vi "ChooseCowlState.vi"(0 "Distance":dbl) -> (1 "A,B,C":string)   [LabVIEW 2019]
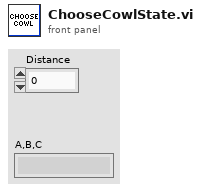
[diagram p1: front panel]
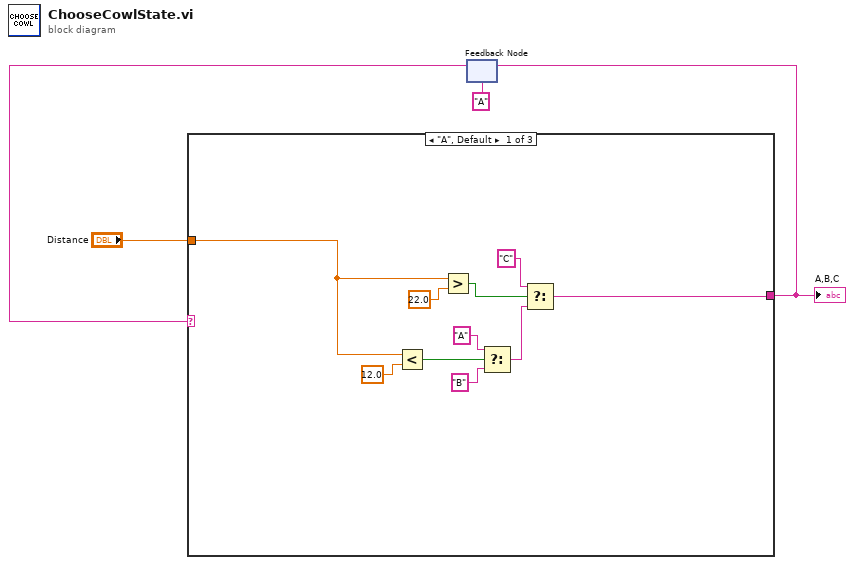
[diagram p0: block diagram]
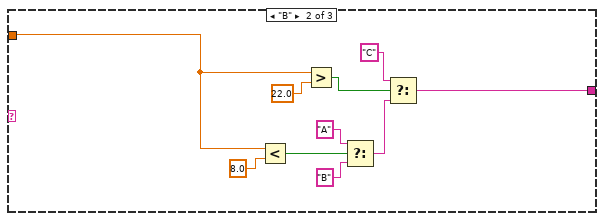
[diagram p2: hidden frame]
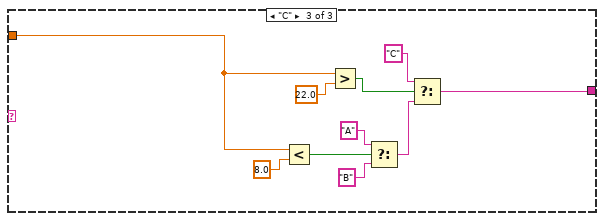
[diagram p3: hidden frame]
diagram:
  n1 = feedback #1("A") -> (w2:string)
  n2 = case shown="\"A\", Default" w2 {
    tunnel: "Distance" -> [w10 w16 w25]
    tunnel: [w5 w17 w26] -> w3
    frame "A", Default {
      n3 = Less?(x=w10, y=12.0) -> (x < y?=w8:bool)
      n4 = Greater?(x=w10, y=22.0) -> (0:w13:bool)
      n5 = Select(t="A", s=w8, f="B") -> (s? t:f=w6:string)
      n6 = Select(t="C", s=w13, f=w6) -> (s? t:f=w5:string)
    }
    frame "B" {
      n7 = Less?(x=w16, y=8.0) -> (x < y?=w19:bool)
      n8 = Greater?(x=w16, y=22.0) -> (0:w23:bool)
      n9 = Select(t="A", s=w19, f="B") -> (s? t:f=w18:string)
      n10 = Select(t="C", s=w23, f=w18) -> (s? t:f=w17:string)
    }
    frame "C" {
      n11 = Less?(x=w25, y=8.0) -> (x < y?=w29:bool)
      n12 = Greater?(x=w25, y=22.0) -> (0:w33:bool)
      n13 = Select(t="A", s=w29, f="B") -> (s? t:f=w27:string)
      n14 = Select(t="C", s=w33, f=w27) -> (s? t:f=w26:string)
    }
  }
  "A,B,C" <- w3
  n15 = feedback-in #1(w3) -> ()
